vi "Read id.vi"(8 "error in (no error)":errorcluster, 11 "Tool Path in":refnum<class "Tool Path.lvclass">) -> (0 "error out":errorcluster, 2 "id":string, 3 "Tool Path out":refnum<class "Tool Path.lvclass">)   [LabVIEW 2019, in "Tool Path.lvclass"]
uses:
  Tool Path.lvclass
  Parse/ParsePaths/Path.lvclass
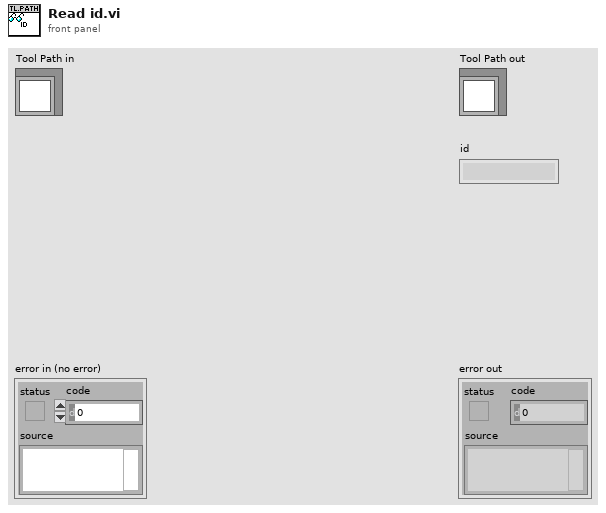
[diagram p1: front panel]
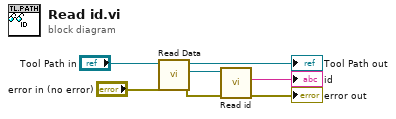
[diagram p0: block diagram]
diagram:
  n1 = call-dynamic "Read Data.vi"("error in (no error)"="error in (no error)", "Tool Path in"="Tool Path in") -> ("error out"=w1:errorcluster, "Path.lvclass"=w7:refnum<class "Path.lvclass">, "Tool Path out"=→"Tool Path out":refnum<class "Tool Path.lvclass">)  [unwired: 7 in]
  n2 = call-dynamic "Read id.vi"("error in (no error)"=w1, "Path in"=w7) -> ("error out"=→"error out":errorcluster, "id"=→"id":string)  [unwired: 7 in, 1 out]
